vi "SubstituteClusterElementByLabel.vi"(8 "error in (no error)":errorcluster, 9 "ElementHierarchy":string[](array[string]), 10 "NewElementValue":variant, 11 "ClusterIn":variant) -> (0 "ErrorOut":errorcluster, 2 "Success?":bool, 3 "UpdatedClusterOut":variant)   [LabVIEW 2020]
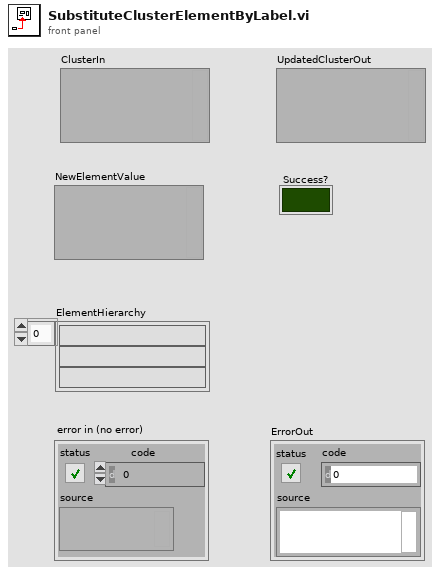
[diagram p1: front panel]
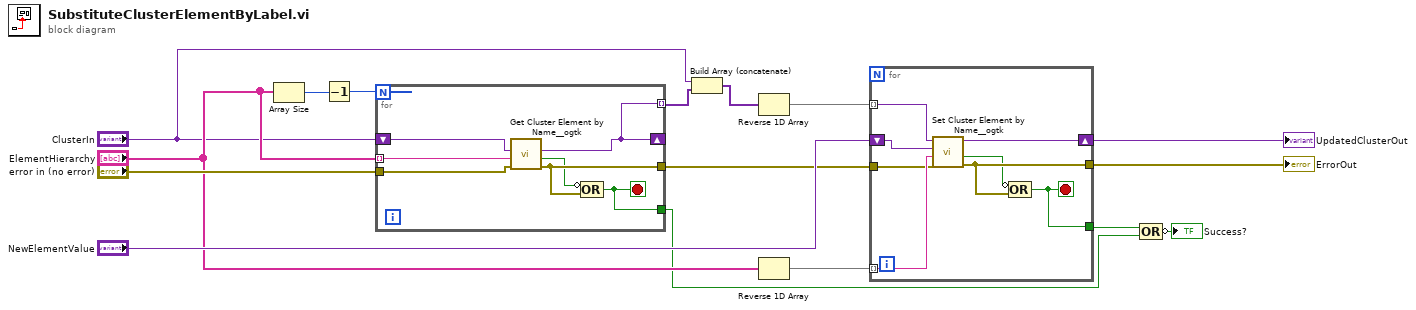
[diagram p0: block diagram]
diagram:
  n1 = Array Size(array="ElementHierarchy") -> (size(s)=w16:i32)
  n2 = Decrement(x=w16) -> (x-1=w14:i32)
  n3 = for {
    N: w14 -> [_]
    tunnel: "ElementHierarchy" -> [w23] mode=indexing
    shift-right: [w21] -> _
    shift-left: "ClusterIn" -> [w22]
    tunnel: [w21] -> w5 mode=indexing
    tunnel: [w19] -> w11
    tunnel: "error in (no error)" -> [w20]
    tunnel: [w17] -> w7
    stop <- w17 stop-if-true
    n4 = call <userlib>:"Get Cluster Element by Name__ogtk.vi"("error in (no error)"=w20, "Element Name"=w23, "Cluster"=w22) -> ("error out"=w19:errorcluster, "found?"=w18:bool, "VElement"=w21:variant)  [unwired: 6 in]
    n5 = Compound Arithmetic op=OR(invert w18, w19) -> (w17:bool)
  }
  n6 = Build Array (concatenate)("ClusterIn", w5) -> (w3:variant[])
  n7 = Reverse 1D Array(array=w3) -> (reversed array=w13:variant[])
  n8 = Reverse 1D Array(array="ElementHierarchy") -> (reversed array=w15:string[])
  n9 = for {
    tunnel: w15 -> [w31] mode=indexing
    tunnel: w13 -> [w28] mode=indexing
    shift-right: [w29] -> w2
    shift-left: "NewElementValue" -> [w30]
    tunnel: w11 -> [w27]
    tunnel: [w26] -> w1
    tunnel: [w24] -> w8
    stop <- w24 stop-if-true
    n10 = call <userlib>:"Set Cluster Element by Name__ogtk.vi"("error in (no error)"=w27, "Element Name (\"\": New Element Data Name)"=w31, "New Element Value"=w30, "Cluster"=w28) -> ("error out"=w26:errorcluster, "found?"=w25:bool, "VCluster out"=w29:variant)  [unwired: 5 in]
    n11 = Compound Arithmetic op=OR(invert w25, w26) -> (w24:bool)
  }
  "UpdatedClusterOut" <- w2
  "ErrorOut" <- w1
  n12 = Compound Arithmetic op=OR(w8, w7) -> (invert →"Success?":bool)
